vi "Photon Canon.vi"(11 "input cluster":T1) -> ()   [LabVIEW 2015]
uses:
  Joystick/ControlsToCommands.ctl
  <vilib>/Rock Robotics/WPI/Relay/WPI_RelayValue.ctl
  References/Refnums.vi
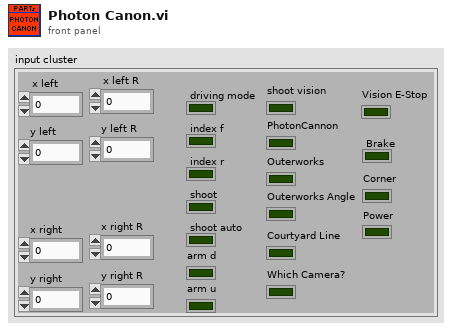
[diagram p1: front panel]
types:
  T1 = typedef "ControlsToCommands.ctl" = cluster{"x left":dbl, "y left":dbl, "x right":dbl, "y right":dbl, "driving mode":bool, "index f":bool, "index r":bool, "shoot":bool, "shoot auto":bool, "arm d":bool, "arm u":bool, "shoot vision":bool, "PhotonCannon":bool, "Outerworks":bool, "Outerworks Angle":bool, "Courtyard Line":bool, "Which Camera?":bool, "Vision E-Stop":bool, "x left R":dbl, "y left R":dbl, "x right R":dbl, "y right R":dbl, "Brake":bool, "Corner":bool, "Power":bool}
  T2 = typedef "WPI_RelayValue.ctl" = enum16{"Off", "On", "Forward", "Reverse"}
  T3 = typedef "WPI_RelayDevRef.ctl" = cluster{"DevStatus":errorcluster, "Relay Channel":T4, "Relay Direction":T5}
  T4 = typedef "FPGA_DIORelayChannel.ctl" = enum8{"Relay 0", "Relay 1", "Relay 2", "Relay 3", "Invalid"}
  T5 = typedef "WPI_RelayDirection.ctl" = enum16{"Both directions", "Forward only", "Reverse only"}
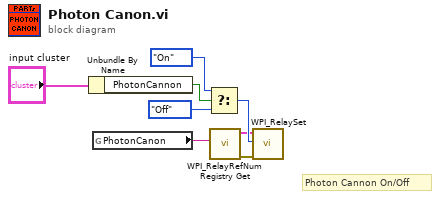
[diagram p0: block diagram]
diagram:
  # "Photon Cannon On/Off"
  n1 = Unbundle By Name("input cluster") -> ("PhotonCannon"=w7:bool)
  n2 = global read "Refnums.vi" "PhotonCanon"() -> (w1:string)
  n3 = Select(t=WPI_RelayValue."On" ("RelayValue"), s=w7, f=WPI_RelayValue."Off" ("RelayValue")) -> (s? t:f=w4:T2)
  n4 = call <vilib>:"WPI_RelayRefNum Registry Get.vi"("refnum name"=w1) -> ("error out"=w2:errorcluster, "RelayDevRef"=w3:T3)  [unwired: 9 in]
  n5 = call <vilib>:"WPI_RelaySet.vi"("error in (no error)"=w2, "RelayValue"=w4, "RelayDevRef"=w3) -> ()  [unwired: 7 in, 2 out]
